vi "Get Bitfile Checksum.vi"(8 "error in (no error)":errorcluster, 11 "ID in":T1 format="%.0x") -> (0 "error out":errorcluster, 1 "Path":string, 2 "MD5":string, 3 "ID out":T1 format="%.0x")   [LabVIEW 2011, in "Sensor Simulation Custom Device.lvlib"]
uses:
  Sensor Simulation Custom Device.lvlib
  <vilib>/NI Veristand/Custom Device API/Custom Device Item Ref.ctl
  NationalInstruments.VeriStand.SystemDefinitionAPI
  <vilib>/Utility/sysdir.llb/System Directory Type.ctl
  <vilib>/NI Veristand/Custom Device Offline API/Custom Device Offline API.lvlib
  <vilib>/NI Veristand/Custom Device API/Custom Device API.lvlib
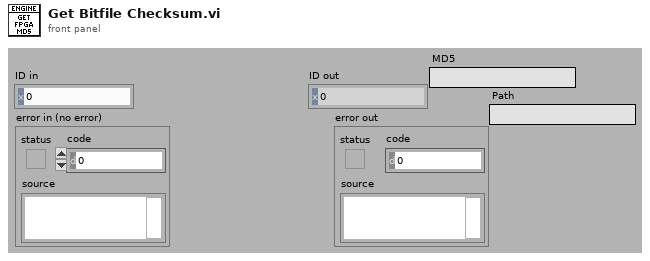
[diagram p1: front panel]
types:
  T1 = typedef "Custom Device API.lvlib/Custom Device Item Ref.ctl" = u64
  T2 = typedef "System Directory Type.ctl" = i32
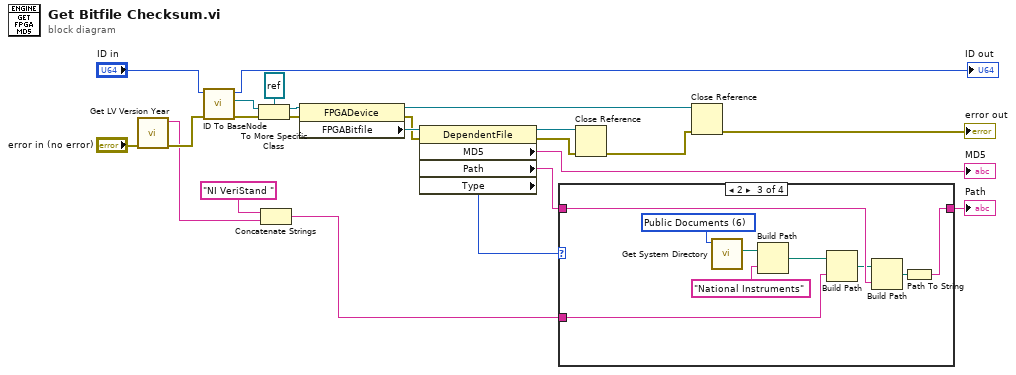
[diagram p0: block diagram]
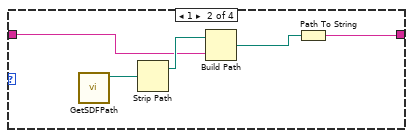
[diagram p3: hidden frame]
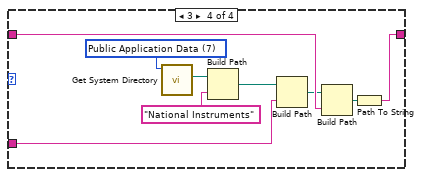
[diagram p4: hidden frame]
diagram:
  n1 = call "Get LV Version Year.vi"("error in (no error)"="error in (no error)") -> ("error out"=w4:errorcluster, "Year"=w2:string)  [unwired: 9 in]
  n2 = call <vilib>:"ID To BaseNode.vi"("error in (no error)"=w4, "ID in"="ID in") -> ("error out"=w21:errorcluster, "BaseNode"=w23:refnum<k24>, "ID out"=→"ID out":u64)  [unwired: 7 in]
  n3 = To More Specific Class(target class=refnum<k24> refnum ("BaseNodeType"), reference=w23, error in=w21) -> (specific class reference=w20:refnum<k24>, error out=w19:errorcluster)
  n4 = Concatenate Strings("NI VeriStand " ("name or relative path"), w2) -> (w1:string)
  n5 = property class="FPGADevice"(reference=w20, error in=w19) -> (reference out=w15:refnum<k24>, error out=w13:errorcluster, "FPGABitfile"=w14:refnum<k24>)
  n6 = property class="DependentFile"(reference=w14, error in=w13) -> (reference out=w11:refnum<k24>, error out=w12:errorcluster, "MD5"=→"MD5":string, "Path"=w6:string, "Type"=w8:i32)
  n7 = case shown="2" w8 {
    tunnel: [w24 w25 w33 w42] -> w7
    tunnel: w6 -> [w24 w27 w35 w44]
    tunnel: w1 -> [_ _ w30 w39]
    frame 0, Default {
    }
    frame 1 {
      n8 = call "GetSDFPath.vi"() -> ("SDF File Path"=w29:path)  [unwired: 10 in, 1 out]
      n9 = Strip Path(path=w29) -> (stripped path=w28:path)  [unwired: 1 out]
      n10 = Build Path(base path=w28, name or relative path=w27) -> (appended path=w26:path)
      n11 = Path To String(path=w26) -> (string=w25:string)
    }
    frame 2 {
      w38 = T2 6 items=["User Home"=0, "User Desktop"=1, "User Documents"=2, "User Application Data"=3, "User Preferences"=4, "User Temporary"=5, "Public Documents"=6, "Public Application Data"=7, "Public Preferences"=8, "Public Cache"=13, "System Core Libraries"=9, "System Installed Libraries"=10, "Application Files"=11, "Boot Volume Root"=12] ("system directory type")
      n12 = call <vilib>:"Get System Directory.vi"("system directory type"=w38) -> ("system directory"=w37:path)  [unwired: 10 in]
      n13 = Build Path(base path=w37, name or relative path="National Instruments") -> (appended path=w31:path)
      n14 = Build Path(base path=w31, name or relative path=w30) -> (appended path=w32:path)
      n15 = Build Path(base path=w32, name or relative path=w35) -> (appended path=w34:path)
      n16 = Path To String(path=w34) -> (string=w33:string)
    }
    frame 3 {
      w47 = T2 7 items=["User Home"=0, "User Desktop"=1, "User Documents"=2, "User Application Data"=3, "User Preferences"=4, "User Temporary"=5, "Public Documents"=6, "Public Application Data"=7, "Public Preferences"=8, "Public Cache"=13, "System Core Libraries"=9, "System Installed Libraries"=10, "Application Files"=11, "Boot Volume Root"=12] ("system directory type")
      n17 = call <vilib>:"Get System Directory.vi"("system directory type"=w47) -> ("system directory"=w46:path)  [unwired: 10 in]
      n18 = Build Path(base path=w46, name or relative path="National Instruments") -> (appended path=w40:path)
      n19 = Build Path(base path=w40, name or relative path=w39) -> (appended path=w41:path)
      n20 = Build Path(base path=w41, name or relative path=w44) -> (appended path=w43:path)
      n21 = Path To String(path=w43) -> (string=w42:string)
    }
  }
  "Path" <- w7
  n22 = Close Reference(reference=w11, error in (no error)=w12) -> (error out=w10:errorcluster)
  n23 = Close Reference(reference=w15, error in (no error)=w10) -> (error out=→"error out":errorcluster)
